vi "Determine Warnings with Case Structure .vi"() -> ()   [LabVIEW 2014]
panel:
  out "Warning Text":string
  out "Warning":bool
  in  "Min Temp":dbl
  in  "Max Temp":dbl
  in  "Current Temp":dbl
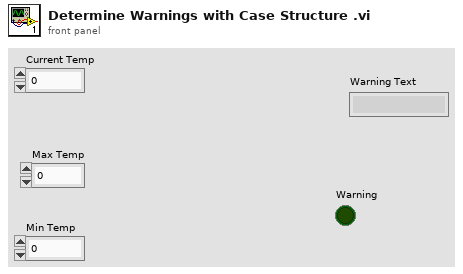
[diagram p1: front panel]
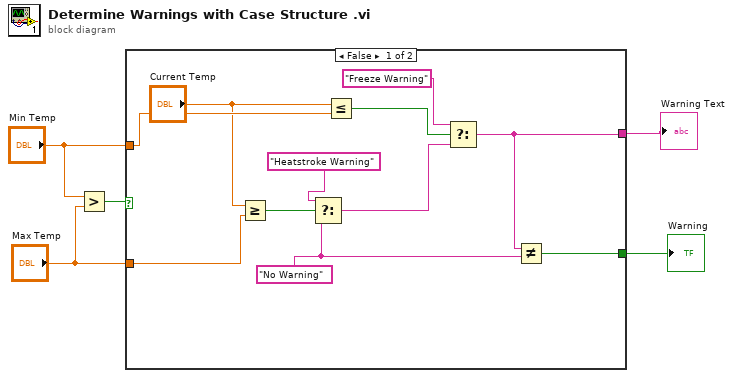
[diagram p0: block diagram]
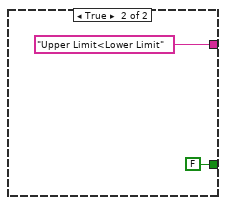
[diagram p2: hidden frame]
diagram:
  n1 = Greater?(x="Min Temp", y="Max Temp") -> (0:w5:bool)
  n2 = case shown="False" w5 {
    tunnel: "Max Temp" -> [w16 _]
    tunnel: "Min Temp" -> [w15 _]
    tunnel: [w7 "Upper Limit<Lower Limit"] -> w2
    tunnel: [w8 FALSE] -> w1
    frame False {
      w6 = "No Warning"
      n3 = Greater Or Equal?(x="Current Temp", y=w16) -> (x >= y?=w12:bool)
      n4 = Select(t="Heatstroke Warning", s=w12, f=w6) -> (s? t:f=w9:string)
      n5 = Less Or Equal?(x="Current Temp", y=w15) -> (x <= y?=w11:bool)
      n6 = Select(t="Freeze Warning", s=w11, f=w9) -> (s? t:f=w7:string)
      n7 = Not Equal?(x=w7, y=w6) -> (x != y?=w8:bool)
    }
    frame True {
    }
  }
  "Warning" <- w1
  "Warning Text" <- w2
